vi "Convert_IMAQtoLVImage.vi"(8 "Error In":errorcluster caption="entrée d'erreur (pas d'erreur)", 11 "IMAQImage In (RGB 32)":T1) -> (0 "Error Out":errorcluster, 1 "cluster de sortie":T2, 2 "Image 2D":picture, 3 "IMAQImage Out":T1)   [LabVIEW 2011]
uses:
  <vilib>/picture/picture.llb/imagedata.ctl
  <vilib>/vision/Image Controls.llb/IMAQ Image.ctl
  Program Files (x86)/National Instruments/LabVIEW 2011/resource/objmgr/IMAQImage.rc
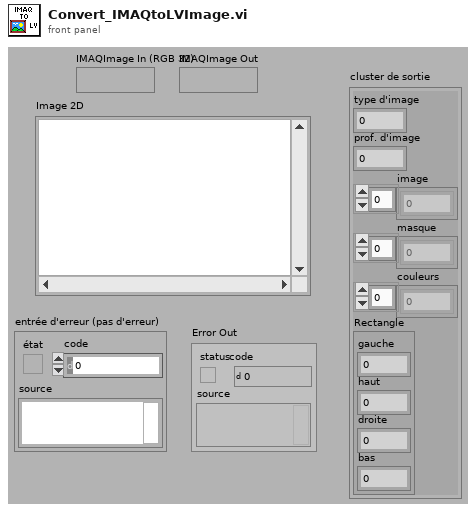
[diagram p1: front panel]
types:
  T1 = typedef "IMAQ Image.ctl" = refnum<image>
  T2 = typedef "imagedata.ctl" = cluster{"image type":i32, "image depth":i32, "image":u8[], "mask":u8[], "colors":u32[], "Rectangle":cluster{"left":i16, "top":i16, "right":i16, "bottom":i16}}
  T3 = cluster{"left":i16, "top":i16, "right":i16, "bottom":i16}
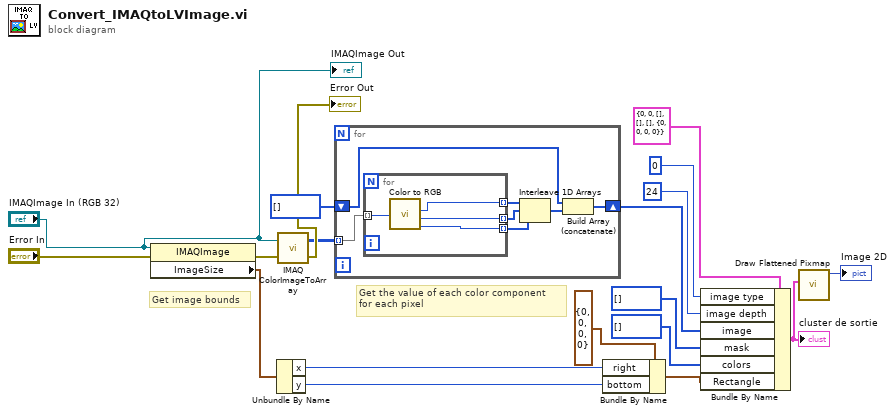
[diagram p0: block diagram]
diagram:
  # "Get the value of each color component\nfor each pixel"
  # "Get image bounds"
  n1 = property class="IMAQImage"(reference="IMAQImage In (RGB 32)", error in="Error In") -> (error out=w6:errorcluster, "ImageSize"=w18:cluster{"x":i32, "y":i32})  [unwired: 1 out]
  n2 = Unbundle By Name(w18) -> ("x"=w13:i32, "y"=w12:i32)
  n3 = call "IMAQ ColorImageToArray"("Image"="IMAQImage In (RGB 32)", "error in (no error)"=w6) -> ("Image Pixels (U32)"=w1:u32[][], "error out"=→"Error Out":errorcluster)  [unwired: 2 in, 1 out]
  n4 = for {
    shift-right: [w24] -> w10
    shift-left: u8[] [] -> [w25]
    tunnel: w1 -> [w23] mode=indexing
    n5 = for {
      tunnel: w23 -> [w30] mode=indexing
      tunnel: [w29] -> w22 mode=indexing
      tunnel: [w28] -> w21 mode=indexing
      tunnel: [w27] -> w20 mode=indexing
      n6 = call <vilib>:"Color to RGB.vi"("Color"=w30) -> ("R"=w29:u8, "G"=w28:u8, "B"=w27:u8)  [unwired: 1 out]
    }
    n7 = Interleave 1D Arrays(w22, w21, w20) -> (w26:u8[])
    n8 = Build Array (concatenate)(w25, w26) -> (w24:u8[])
  }
  n9 = Bundle By Name(cluster=T3 {"left"=0, "top"=0, "right"=0, "bottom"=0} ("Rectangle"), "right"=w13, "bottom"=w12) -> (w17:T3)
  n10 = Bundle By Name(cluster=T2 {"image type"=0, "image depth"=0, "image"=[], "mask"=[], "colors"=[], "Rectangle"={"left"=0, "top"=0, "right"=0, "bottom"=0}} ("image data"), "image type"=0, "image depth"=24 ("Bit Depth (0)"), "image"=w10, "mask"=u8[] [], "colors"=u32[] [], "Rectangle"=w17) -> (w8:T2)
  "cluster de sortie" <- w8
  n11 = call <vilib>:"Draw Flattened Pixmap.vi"("image data"=w8) -> ("new picture"=→"Image 2D":picture)  [unwired: 8 in]
  "IMAQImage Out" <- "IMAQImage In (RGB 32)"
